vi "trialrunner.vi"() -> ()   [LabVIEW 2012]
uses:
  testing/log_event.ctl
  Experiment info.ctl
  testing/mode_conrols.ctl
  testing/ui_override_opts.ctl
  testing/control_selector.ctl
  initialization/micron_globals.vi
  <vilib>/Utility/xml.llb/Read From XML File(array).vi
panel:
  out "Actuate":bool
  out "Mode controls":T1
  in  "Allow skipping":bool
  in  "error in":errorcluster
  in  "Data path":string="c:\\data\\trials\\"
  out "Warning":bool
  out "Error":bool
  out "Retake":bool
  in  "Config name":string="trial"
  in  "Result data decimate":i32=5
  out "Start time":u32
  out "Prompt number":i32
  out "File exists":bool
  in  "Completed Trial Index":i32
  out "Information":string
  in  "New Experiment":bool
  out "Num Trials":i32
  in  "Back":bool
  in  "Next":bool
  in  "Subject Information":T2={" Subject"=-1, " Experiment"=1}
  in  "Trial Index":i32
  out "Trial status":T3[](array[typedef]) {"Timestamp" format="%<%.3X>T"}
  in  "Stop trial":bool caption="Stop"
  in  "Start":bool
  out "Run/stop":bool
  out "File name":path
  out "Save trace":bool
  in  "stop":bool
  # "Subject Information"
  # "Trial Management"
  # "m"
  # "Micron \nTrial \nManager"
  # "Authorized Personnel Only"
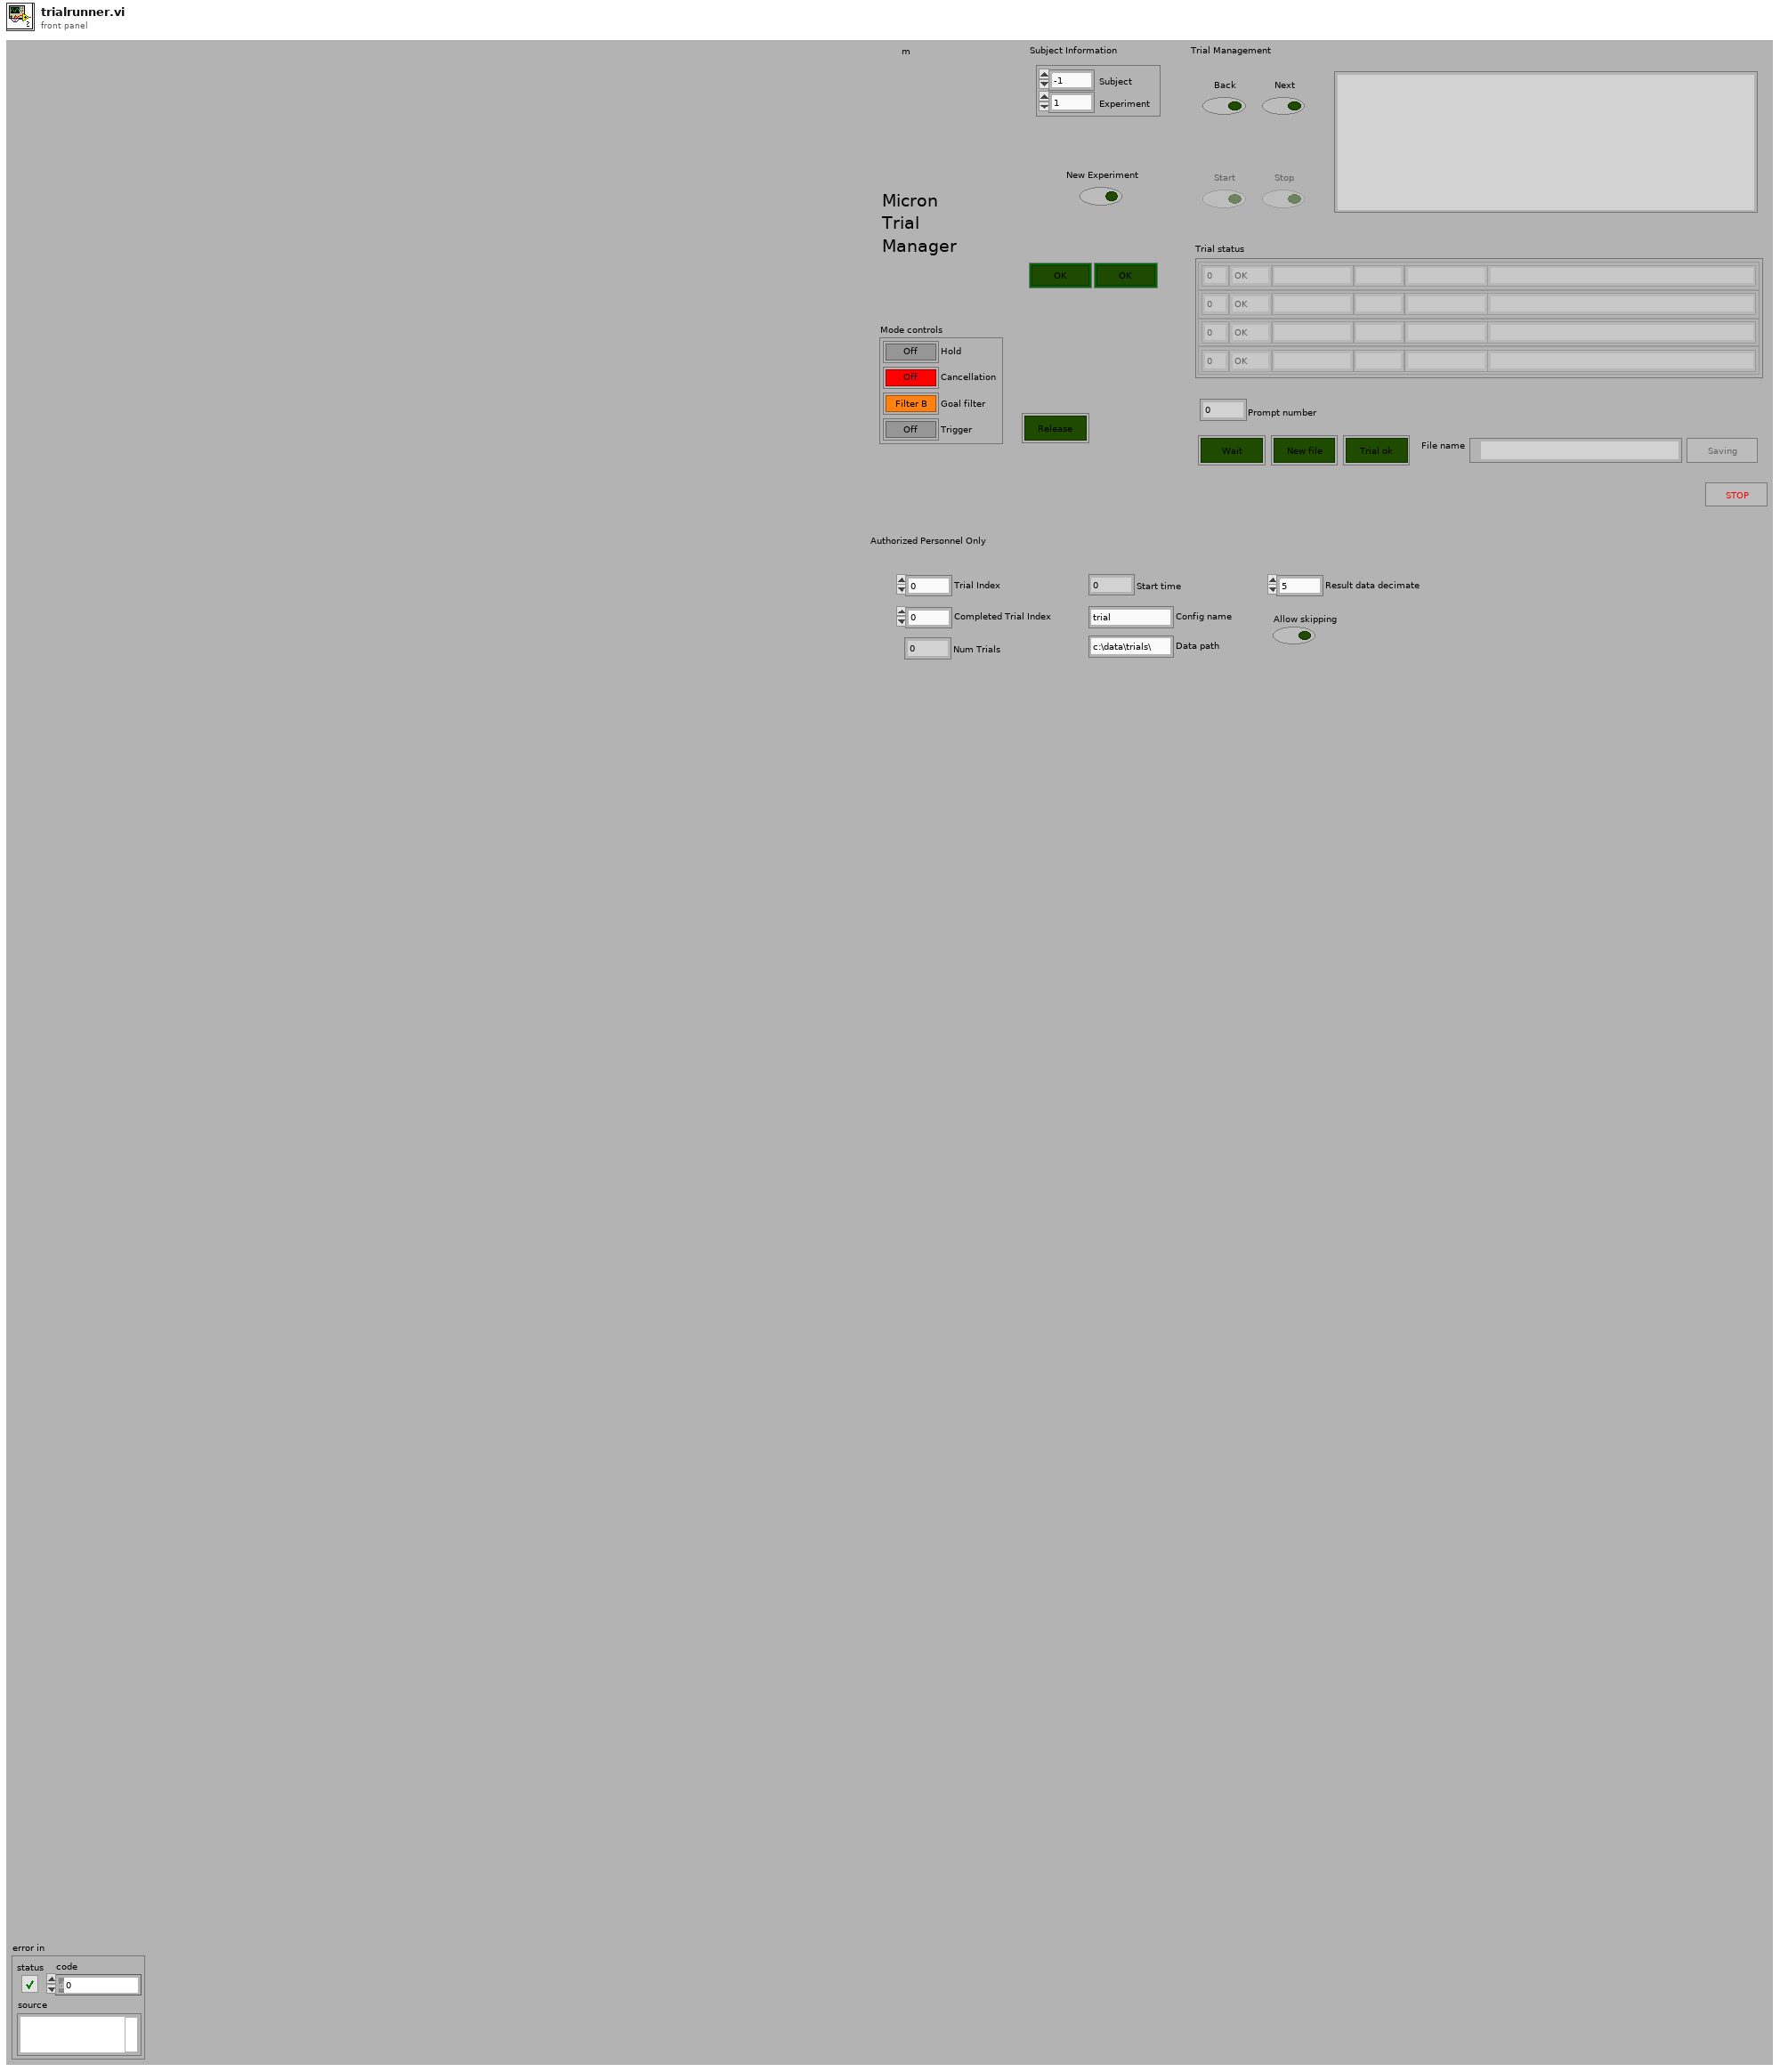
[diagram p1: front panel]
types:
  T1 = typedef "mode_conrols.ctl" = cluster{"Hold":bool, "Cancellation":bool, "Goal filter":bool, "Trigger":bool}
  T2 = typedef "Experiment info.ctl" = cluster{" Subject":i32, " Experiment":i32}
  T3 = typedef "log_event.ctl" = cluster{"Facility ID":i32, "Severity":enum16{"OK", "Debug", "Warn", "Error"}, "Timestamp":timestamp, "Facility":string, "State":string, "Message":string}
  T4 = typedef "ui_override_opts.ctl" = cluster{"Triggering":bool, "Parameters":bool, "Stimulus":bool, "Calibration":bool, "Modes":bool}
  T5 = typedef "Micron params.ctl" = cluster{"Stimulus":T6, "Goal Filter A":T8, "Mode controls":T1, "Manipulator type":enum16{"Current piezo", "Voltage piezo"}, "Manipulator calibration":T9, "Network":T11, "Goal Filter B":T8, "Cancellation":T12, "Transition time":sgl, "Estimation":T14}
  T6 = typedef "stimulus.ctl" = cluster{"Type":enum16{"Off", "Step", "Sine", "Triangle", "Arbitrary"}, "Phase":dbl, "Amplitude":sgl[], "Injection point":T7, "Closed loop":bool, "Offset":sgl[], "Tip -> world":bool, "Frequency":dbl, "Length":dbl}
  T7 = typedef "injection_point.ctl" = enum16{"Total pose", "V limiter", "Goal ", "Link position", "KF link position", "Inverse kin", "Link goal", "Link error", "Controller", "Output", "Drive", "Light"}
  T8 = typedef "goal_loop_parms.ctl" = cluster{"Speedup max":sgl, "Speedup thresh":sgl, "Speedup nonlin":sgl, "Filters":cluster{"Lower Fc":sgl, "Lower Q":sgl, "Scale factor":sgl, "Upper Fc":sgl, "Upper Q":sgl, "V limit":sgl, "V limit range":sgl}[]}
  T9 = typedef "manipulator_cal.ctl" = cluster{"Tool offsets":sgl[][], "Tip light calibration":T10, "Handle light calibration":T10, "Base pivots":sgl[][], "Output pivots":sgl[][], "Length center":sgl, "Workspace height":sgl[], "Workspace diameter":sgl[], "Linearization":sgl[][], "Stack travel":sgl, "Saturation pos":sgl, "Inverse filters":cluster{"filter structure":enum32{"IIR 2nd Order", "IIR 4th Order"}, "Reverse Coefficients":dbl[], "Forward Coefficients":dbl[]}[]}
  T10 = typedef "probe_calibration.ctl" = sgl[][]
  T11 = typedef "network_params.ctl" = cluster{"Remote Host":string, "Send Status":bool, "Send Port":u16, "Recv Commands":bool, "Recv Port":u16}
  T12 = typedef "sq_control_params.ctl" = cluster{"KP":T13, "KI":sgl, "KD":T13, "Max vel":sgl, "Max acc":sgl, "Int error limit":sgl, "RCM gain":sgl, "Bypass":bool, "Degraded gain":sgl}
  T13 = typedef "decoupled_gain.ctl" = cluster{"XY":sgl, "Rxy":sgl, "Z":sgl, "Rz":sgl}
  T14 = typedef "estimation_controls.ctl" = cluster{"Link":cluster{"Measure noise":dbl[], "Process noise":dbl[], "Alt process noise":dbl[], "Alt turnoff cycles":i32, "Innovation limit":dbl[], "Residue threshold":dbl, "Enable":bool}, "Handle":cluster{"Measure noise":dbl[], "Process noise":dbl[], "State limits":dbl[], "Innovation limit":dbl[], "Prediction Lookahead":sgl, "Enable":bool}}
  T15 = typedef "Rendezvous RefNum" = refnum<k1>
  T16 = typedef "control_selector.ctl" = cluster{"Selection":enum32{"No Selection", "Left", "Middle", "Right"}, "Mode":enum16{"Up", "Down", "Toggle", "Pulse", "Always", "Never"}}
  T17 = enum8{"Enabled", "Disabled", "Disabled and Grayed Out"}
  T18 = typedef "micron_config.ctl" = cluster{"rt fifo":refnum<k33>, "Analog output task":refnum<k21>, "Analog output task 2":refnum<k21>, "Stimulus AO task":refnum<k21>, "Low-rate AIN task":refnum<k21>, "Pedal out task":refnum<k21>, "Pedal in task":refnum<k21>, "Loop timing source":string, "Relay out task":refnum<k21>, "Send UDP Conn":refnum<k16>, "Recv UDP Conn":refnum<k16>, "Host Addr":dbl, "I2C interface":T19, "trace_start notifier":refnum<notifier>, "trace_done notifier":refnum<notifier>, "ASAP FIFO":refnum<k33>}
  T19 = typedef "i2c_interface.ctl" = cluster{"FPGA VI Reference":T20}
  T20 = typedef "fpga_reference.ctl" = refnum<k20>
  T21 = typedef "trial_condition.ctl" = cluster{"Type":enum16{"Undefined", "Start", "Normal", "Rest", "Done"}, "Task":u16, "Code":string, "Duration":dbl, "Prompts":u16, "Mode controls":T1, "Variable":bool, "Hold":bool}
  T22 = enum16{"Undefined", "Start", "Normal", "Rest", "Done"}
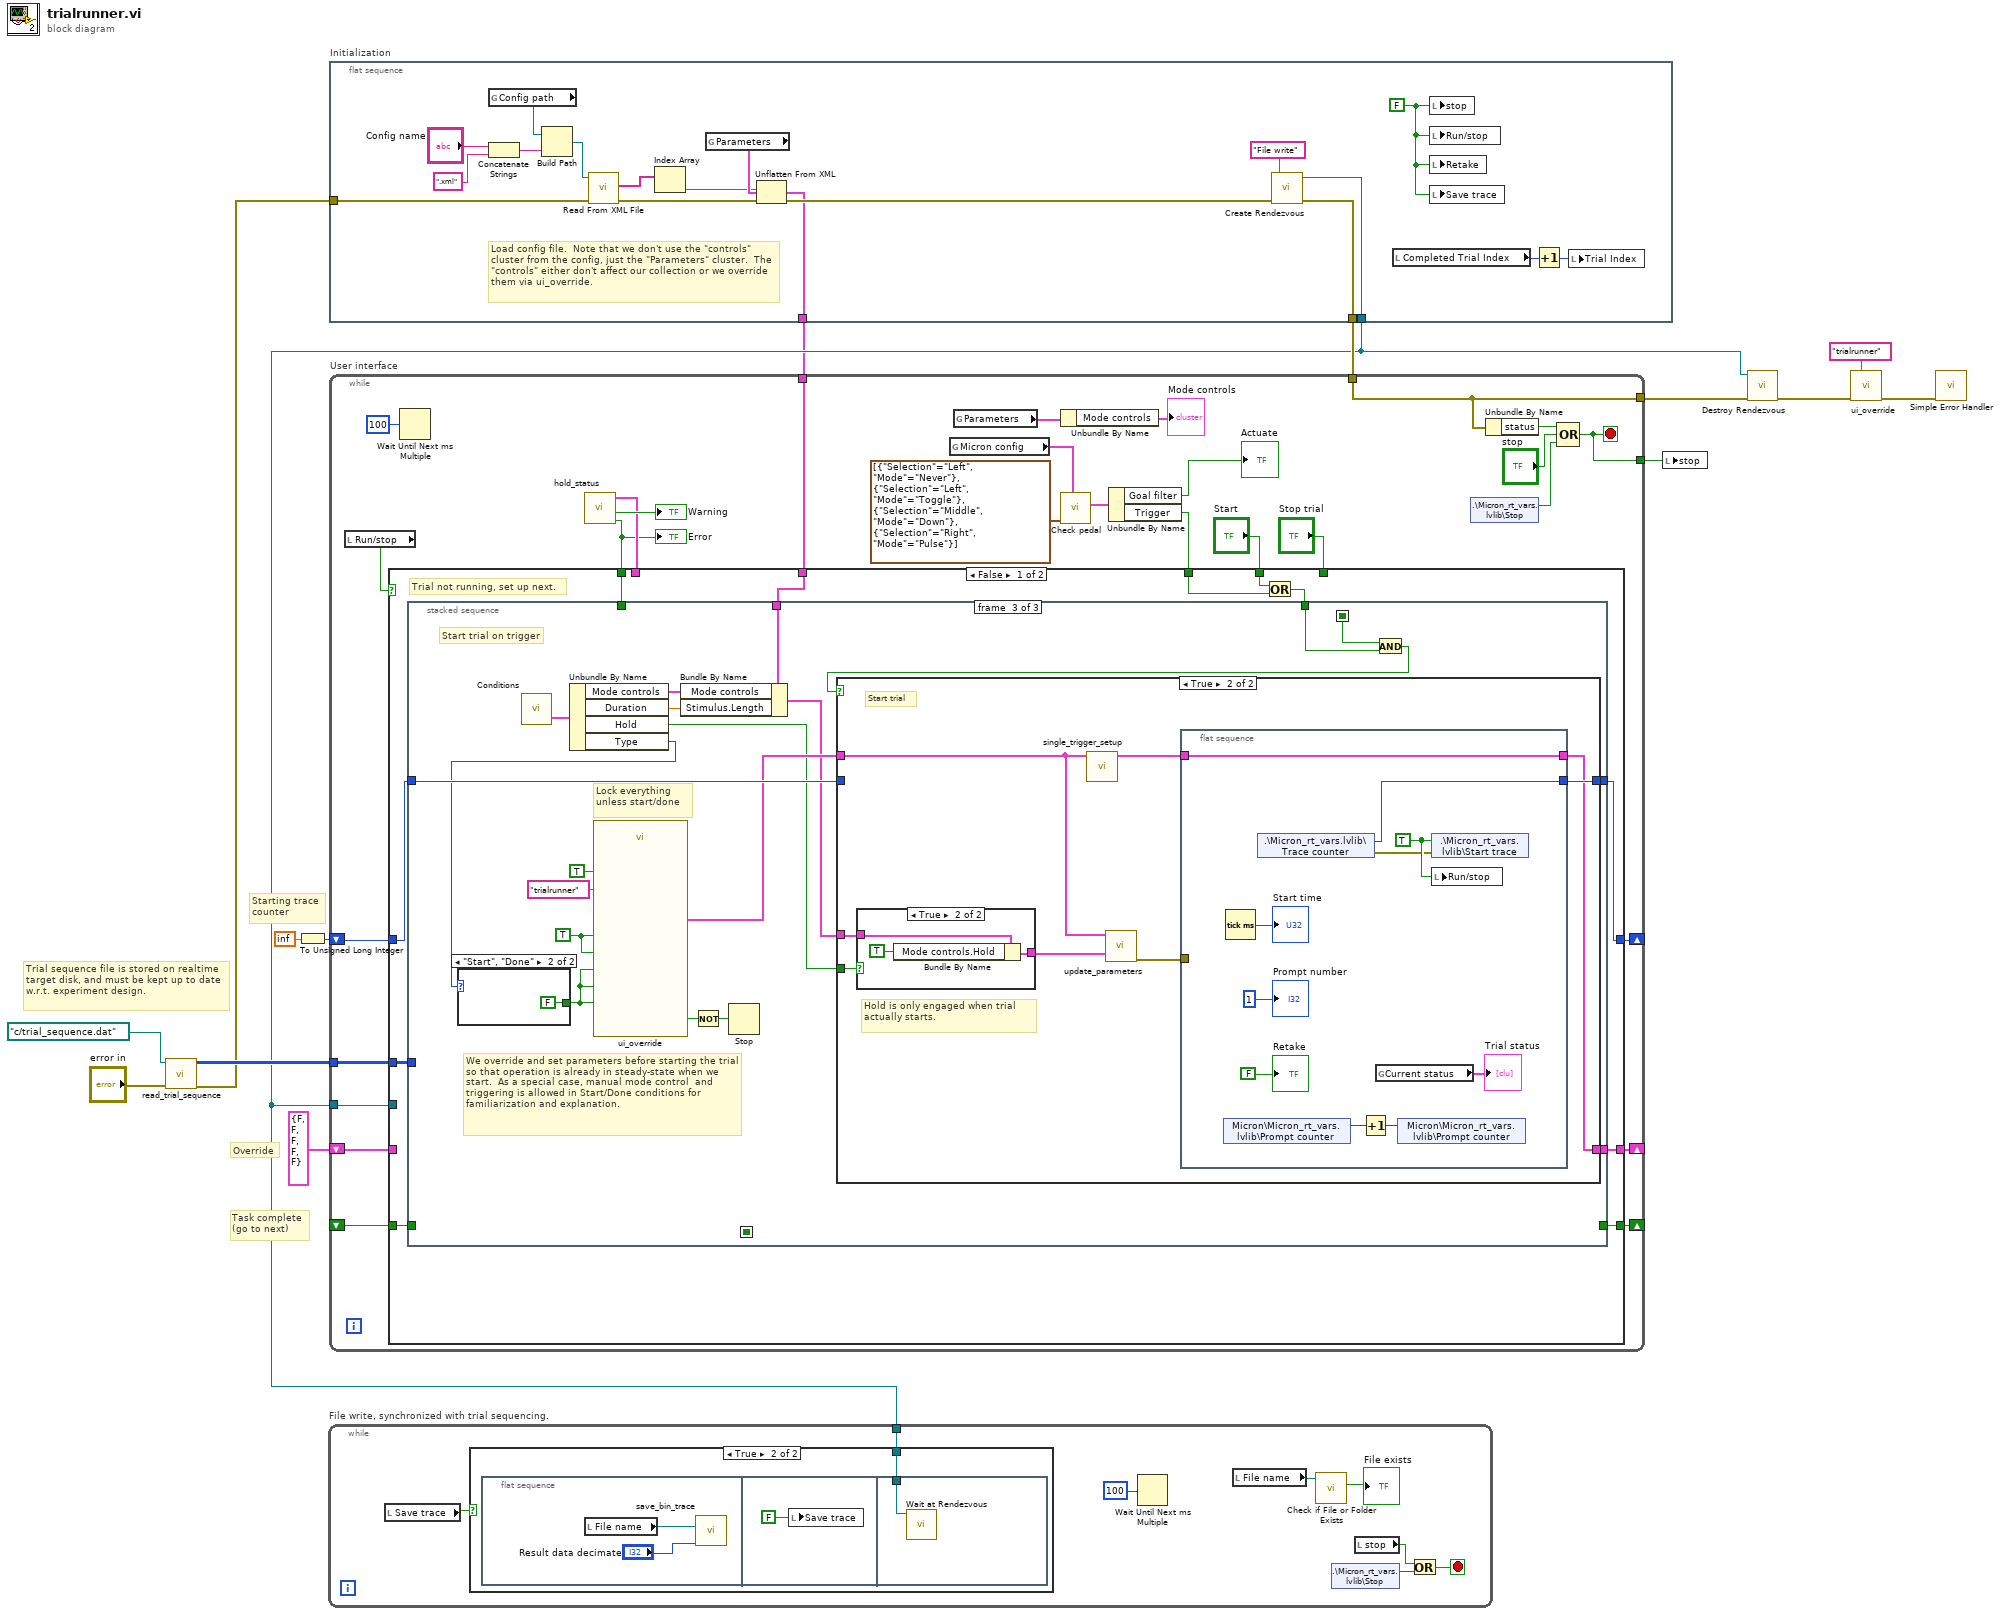
[diagram p0: block diagram]
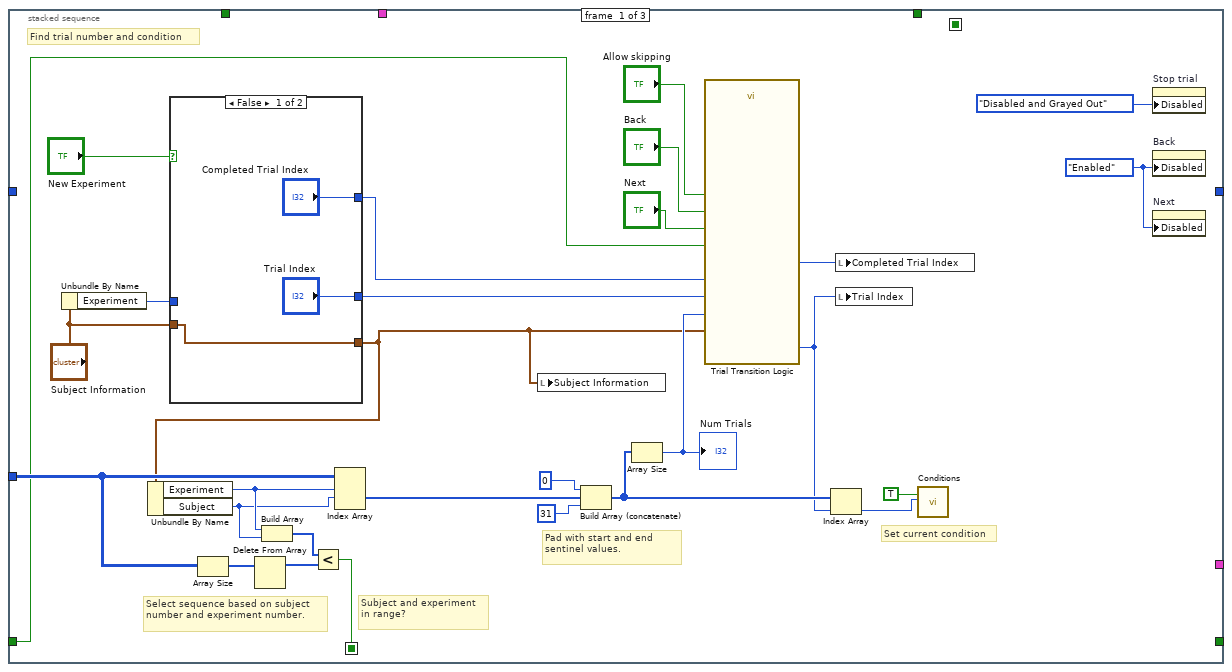
[diagram p2: hidden frame]
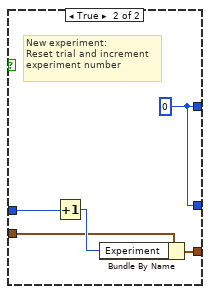
[diagram p3: hidden frame]
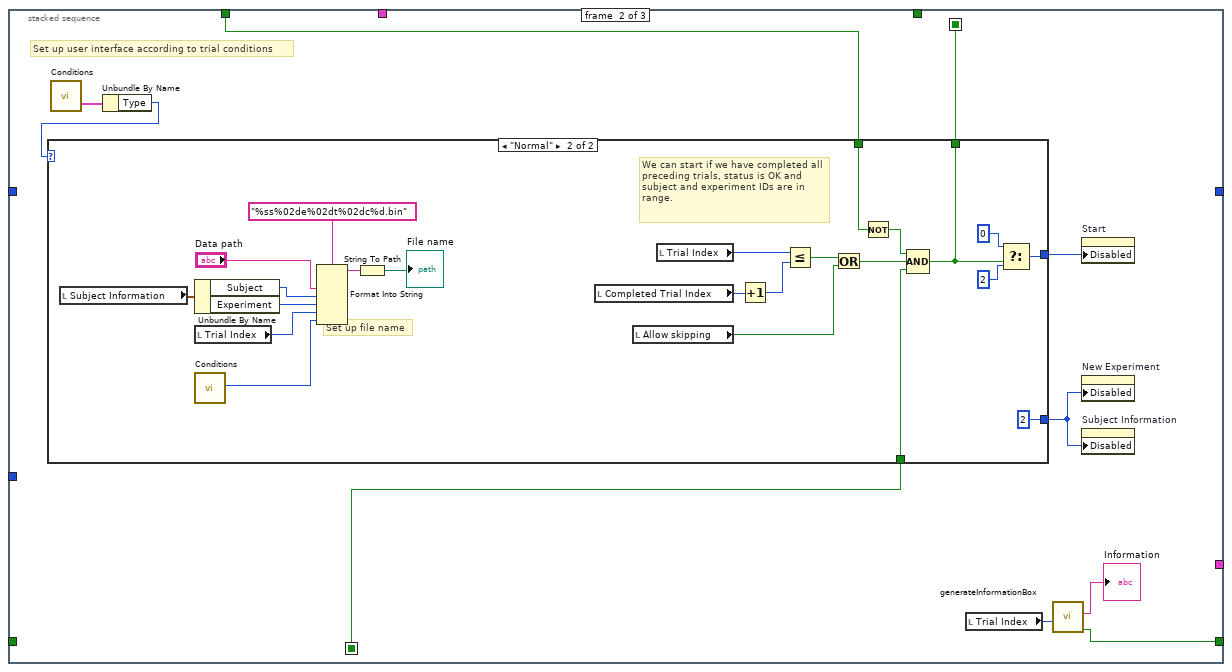
[diagram p4: hidden frame]
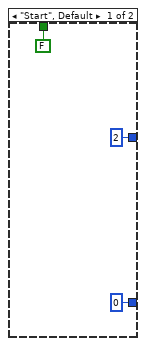
[diagram p5: hidden frame]
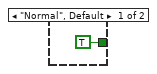
[diagram p6: hidden frame]
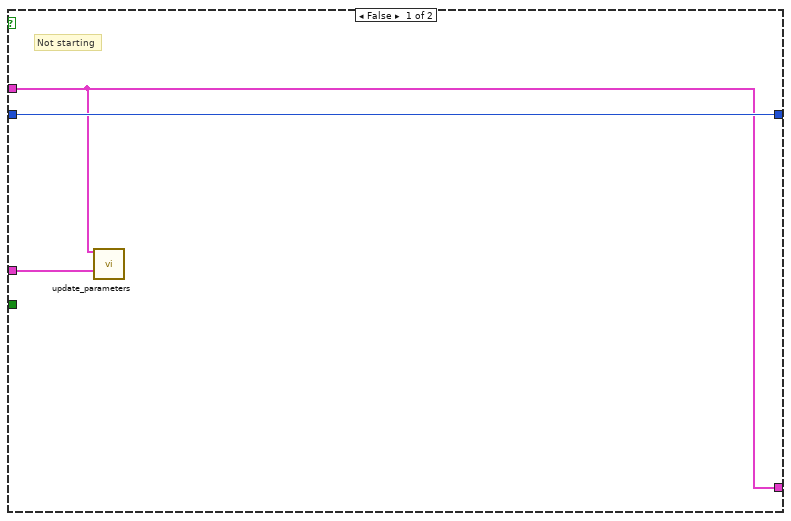
[diagram p7: hidden frame]
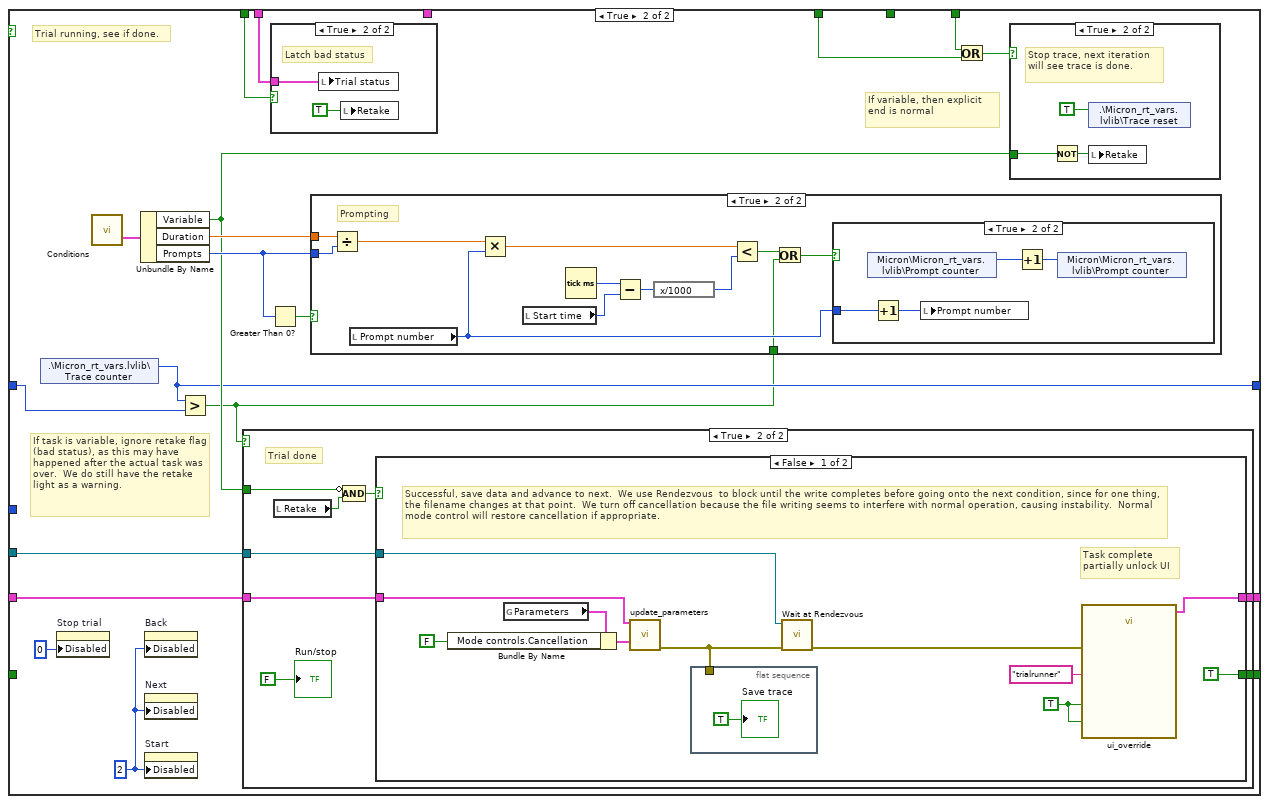
[diagram p9: hidden frame]
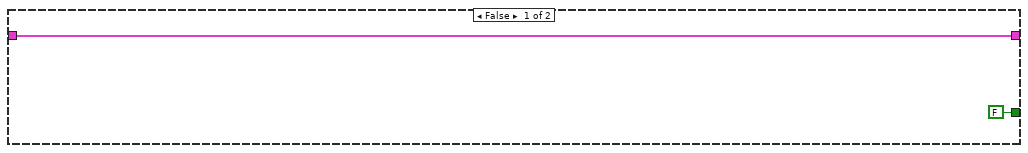
[diagram p13: hidden frame]
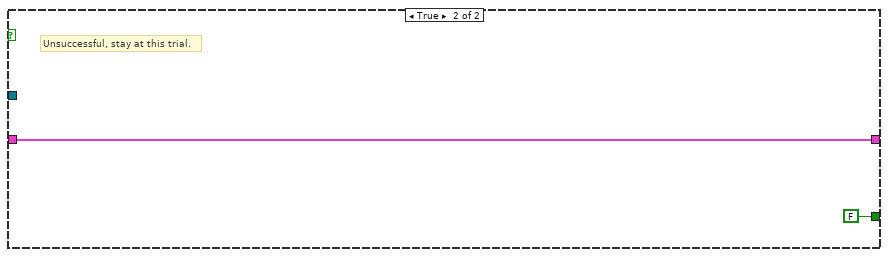
[diagram p14: hidden frame]
diagram:
  # "Override"
  # "Starting trace \ncounter"
  # "Task complete\n(go to next)"
  # "Trial sequence file is stored on realtime target disk, and must be kept up to date w.r.t. experiment design."
  n1 = call "read_trial_sequence.vi"("error in (no error)"="error in", "file path"=path "c:/trial_sequence.dat" ("file path (dialog if empty)")) -> ("error out"=w4:errorcluster, "Array"=w15:i32[][][])  [unwired: 8 in]
  n2 = To Unsigned Long Integer(number=inf) -> (unsigned 32bit integer=w1:u32)
  n3 = while "File write, synchronized with trial sequencing." {
    tunnel: w12 -> [w22]
    stop <- w16 stop-if-true
    n4 = local read "Save trace"() -> (w23:bool)
    n5 = case shown="True" w23 {
      tunnel: w22 -> [_ w24]
      frame False {
      }
      frame True {
        n6 = flat-sequence {
          tunnel: w24 -> [w28]
          frame #0 {
            n7 = local read "File name"() -> (w26:path)
            n8 = call "save_bin_trace.vi"("Decimate"="Result data decimate", "File path"=w26) -> ()  [unwired: 10 out]
          }
          frame #1 {
            n9 = local write "Save trace"(FALSE ("Save trace")) -> ()
          }
          frame #2 {
            n10 = call <vilib>:"Wait at Rendezvous.vi"("rendezvous"=w28) -> ()  [unwired: 2 in, 5 out]
          }
        }
      }
    }
    n11 = Wait Until Next ms Multiple(millisecond multiple=u32 100) -> ()  [unwired: 1 out]
    n12 = local read "File name"() -> (w20:path)
    n13 = call <vilib>:"Check if File or Folder Exists.vi"("path"=w20) -> ("file or folder exists?"=→"File exists":bool)  [unwired: 1 in, 9 out]
    n14 = shared-variable ".\\Micron_rt_vars.lvlib\\Stop"() -> (w18:bool)  [unwired: 2 out]
    n15 = local read "stop"() -> (w17:bool)
    n16 = Or(x=w17, y=w18) -> (x .or. y?=w16:bool)
  }
  n17 = flat-sequence "Initialization" {
    tunnel: [w45] -> w14
    tunnel: [w44] -> w12
    tunnel: [w31] -> w11
    tunnel: w4 -> [w29]
    frame #0 {
      w30 = FALSE ("Run/stop")
      # "Load config file.  Note that we don't use the \"controls\"  cluster from the config, just the \"Parameters\" cluster.  The \"controls\" either don't affect our collection or we override them via ui_override."
      n18 = global read "micron_globals.vi" "Config path"() -> (w39:path)
      n19 = Concatenate Strings("Config name", ".xml" ("string")) -> (w38:string)
      n20 = Build Path(base path=w39, name or relative path=w38) -> (appended path=w41:path)
      n21 = call-poly <vilib>:"Read From XML File.vi"("error in (no error)"=w29, "XML File Path"=w41) -> ("error out"=w33:errorcluster, "XML Elements"=w35:string[])  [unwired: 8 out]
      n22 = Index Array(array=w35) -> (element=w34:string)  [unwired: 1 in]
      n23 = global read "micron_globals.vi" "Parameters"() -> (w36:T5)
      n24 = Unflatten From XML(xml string=w34, type=w36, error in (no error)=w33) -> (value=w31:T5, error out=w32:errorcluster)
      n25 = call <vilib>:"Create Rendezvous.vi"("error in (no error)"=w32, "name (unnamed)"="File write") -> ("error out"=w45:errorcluster, "rendezvous"=w44:T15)  [unwired: 1 in, 3 out]
      n26 = local read "Completed Trial Index"() -> (w43:i32)
      n27 = local write "stop"(w30) -> ()
      n28 = local write "Run/stop"(w30) -> ()
      n29 = local write "Retake"(w30) -> ()
      n30 = local write "Save trace"(w30) -> ()
      n31 = Increment(x=w43) -> (x+1=w42:i32)
      n32 = local write "Trial Index"(w42) -> ()
    }
  }
  n33 = while "User interface" {
    tunnel: [w55] -> w13
    tunnel: w14 -> [w55]
    shift-right: [w69] -> _
    shift-left: w1 -> [w68]
    tunnel: w15 -> [w67]
    tunnel: w12 -> [w65]
    shift-right: [w63] -> _
    shift-left: _ -> [w62]
    tunnel: w11 -> [w58]
    shift-right: [w57] -> _
    shift-left: T4 {"Triggering"=FALSE, "Parameters"=FALSE, "Stimulus"=FALSE, "Calibration"=FALSE, "Modes"=FALSE} ("Override") -> [w56]
    tunnel: [w50] -> w7
    stop <- w50 stop-if-true
    n34 = local read "Run/stop"() -> (w71:bool)
    n35 = Wait Until Next ms Multiple(millisecond multiple=u32 100) -> ()  [unwired: 1 out]
    n36 = call "hold_status.vi"() -> ("Error"=w59:bool, "Warning"=→"Warning":bool, "Hold status"=w60:T3[])  [unwired: 9 in]
    "Error" <- w59
    n37 = global read "micron_globals.vi" "Micron config"() -> (w54:T18)
    n38 = global read "micron_globals.vi" "Parameters"() -> (w49:T5)
    n39 = Unbundle By Name(w49) -> ("Mode controls"=→"Mode controls":T1)
    n40 = call "Check pedal.vi"("Micron config"=w54, "Pedal selector"=T16[] [{"Selection"=enum."Left", "Mode"=enum."Never"}, {"Selection"=enum."Left", "Mode"=enum."Toggle"}, {"Selection"=enum."Middle", "Mode"=enum."Down"}, {"Selection"=enum."Right", "Mode"=enum."Pulse"}]) -> ("New mode controls"=w53:T1)  [unwired: 1 in, 8 out]
    n41 = Unbundle By Name(w53) -> ("Goal filter"=→"Actuate":bool, "Trigger"=w52:bool)
    n42 = case shown="False" w71 {
      tunnel: [w81 w206] -> w69
      tunnel: w68 -> [w78 w223]
      tunnel: "Start" -> [w83 _]
      tunnel: "Stop trial" -> [_ w220]
      tunnel: w67 -> [w85 _]
      tunnel: w52 -> [w84 w218]
      tunnel: w65 -> [_ w217]
      tunnel: [w80 w212] -> w63
      tunnel: w62 -> [w79 _]
      tunnel: w60 -> [_ w209]
      tunnel: w59 -> [w75 w210]
      tunnel: w58 -> [w77 _]
      tunnel: [w76 w207] -> w57
      tunnel: w56 -> [_ w208]
      frame False {
        # "Trial not running, set up next."
        n43 = Or(x=w83, y=w84) -> (x .or. y?=w82:bool)
        n44 = stacked-sequence {
          seq-local: [_ w124 _] -> [_ _ w177]
          seq-local: [w88 _ _] -> [_ w122 _]
          tunnel: w82 -> [_ _ w176]
          tunnel: w85 -> [w101 _ _]
          tunnel: [_ _ w174] -> w81
          tunnel: [_ w125 _] -> w80
          tunnel: w79 -> [w98 _ _]
          tunnel: w78 -> [_ _ w173]
          tunnel: w77 -> [_ _ w163]
          tunnel: [_ _ w172] -> w76
          tunnel: w75 -> [_ w123 _]
          frame #0 {
            w93 = T17."Enabled" ("Disabled")
            # "Subject and experiment in range?"
            # "Set current condition"
            # "Find trial number and condition"
            # "Pad with start and end sentinel values."
            # "Select sequence based on subject number and experiment number."
            n45 = Unbundle By Name("Subject Information") -> ("Experiment"=w104:i32)
            n46 = case shown="False" "New Experiment" {
              tunnel: w104 -> [_ w121]
              tunnel: "Subject Information" -> [w116 w119]
              tunnel: ["Trial Index" w117] -> w103
              tunnel: [w116 w118] -> w99
              tunnel: ["Completed Trial Index" w117] -> w96
              frame False {
              }
              frame True {
                w117 = 0 ("trialIndex")
                # "New experiment:\nReset trial and increment \nexperiment number"
                n47 = Increment(x=w121) -> (x+1=w120:i32)
                n48 = Bundle By Name(cluster=w119, "Experiment"=w120) -> (w118:T2)
              }
            }
            n49 = Unbundle By Name(w99) -> ("Experiment"=w92:i32, "Subject"=w87:i32)
            n50 = Array Size(array=w101) -> (size(s)=w91:i32[])
            n51 = Delete From Array(array=w91) -> (array with subset deleted=w90:i32[])  [unwired: 2 in, 1 out]
            n52 = Build Array(w92, w87) -> (w89:i32[])
            n53 = Less?(x=w89, y=w90) -> (x < y?=w88:bool)
            n54 = Index Array(array=w101, index (dim 0)=w92, index (dim 1)=w87) -> (element=w110:i32[])  [unwired: 1 in]
            n55 = local write "Subject Information"(w99) -> ()
            n56 = Build Array (concatenate)(0 ("element"), w110, 31 ("element")) -> (w107:i32[])
            n57 = Array Size(array=w107) -> (size(s)=w100:i32)
            "Num Trials" <- w100
            n58 = call "Trial Transition Logic.vi"("Completed Trial Index"=w96, "Allow skipping"="Allow skipping", "Old trial index"=w103, "Back"="Back", "Subject Information"=w99, "Num Trials"=w100, "Task complete"=w98, "Next"="Next") -> ("New Completed Trial Index"=w95:i32, "New trial index"=w102:i32)  [unwired: 2 out]
            n59 = Index Array(array=w107, index=w102) -> (element=w113:i32)
            n60 = local write "Completed Trial Index"(w95) -> ()
            n61 = local write "Trial Index"(w102) -> ()
            n62 = call "Conditions.vi"("Set current"=TRUE, "New condition code"=w113) -> ()  [unwired: 18 out]
            n63 = property on="Stop trial" class="Bool"("Disabled"=T17."Disabled and Grayed Out") -> ()  [unwired: 2 in, 2 out]
            n64 = property on="Back" class="Bool"("Disabled"=w93) -> ()  [unwired: 2 in, 2 out]
            n65 = property on="Next" class="Bool"("Disabled"=w93) -> ()  [unwired: 2 in, 2 out]
          }
          frame #1 {
            # "Set up user interface according to trial conditions"
            n66 = call "Conditions.vi"() -> ("Current condition"=w131:T21)  [unwired: 2 in, 17 out]
            n67 = Unbundle By Name(w131) -> ("Type"=w126:T22)
            n68 = case shown="\"Normal\"" w126 {
              tunnel: [u8 2 ("Disabled") w155] -> w130
              tunnel: [u8 0 ("Disabled") u8 2 ("Disabled")] -> w129
              tunnel: [FALSE w143] -> w124
              tunnel: w123 -> [_ w142]
              tunnel: w122 -> [_ w138]
              frame "Start", Default {
              }
              frame "Normal" {
                # "Set up file name"
                # "We can start if we have completed all preceding trials, status is OK and subject and experiment IDs are in range."
                n69 = local read "Subject Information"() -> (w150:T2)
                n70 = Unbundle By Name(w150) -> ("Subject"=w140:i32, "Experiment"=w145:i32)
                n71 = local read "Trial Index"() -> (w147:i32)
                n72 = call "Conditions.vi"() -> ("Condition code"=w148:i32)  [unwired: 2 in, 17 out]
                n73 = Format Into String(format string="%ss%02de%02dt%02dc%d.bin", "Data path", w140, w145, w147, w148) -> (resulting string=w149:string)  [unwired: 2 in, 1 out]
                n74 = String To Path(string=w149) -> (path=→"File name":path)
                n75 = local read "Completed Trial Index"() -> (w144:i32)
                n76 = local read "Allow skipping"() -> (w135:bool)
                n77 = local read "Trial Index"() -> (w153:i32)
                n78 = Increment(x=w144) -> (x+1=w154:i32)
                n79 = Less Or Equal?(x=w153, y=w154) -> (x <= y?=w137:bool)
                n80 = Or(x=w137, y=w135) -> (x .or. y?=w136:bool)
                n81 = Not(x=w142) -> (.not. x?=w141:bool)
                n82 = Compound Arithmetic op=AND(w141, w136, w138) -> (w143:bool)
                n83 = Select(t=u8 0, s=w143, f=u8 2 ("t")) -> (s? t:f=w155:u8)
              }
            }
            n84 = local read "Trial Index"() -> (w127:i32)
            n85 = call "generateInformationBox.vi"("Trial Index"=w127) -> ("Break over"=w125:bool, "Information Box"=→"Information":string)  [unwired: 4 in, 5 out]
            n86 = property on="Start" class="Bool"("Disabled"=w130) -> ()  [unwired: 2 in, 2 out]
            n87 = property on="New Experiment" class="Bool"("Disabled"=w129) -> ()  [unwired: 2 in, 2 out]
            n88 = property on="Subject Information" class="Clust (strict)"("Disabled"=w129) -> ()  [unwired: 2 in, 2 out]
          }
          frame #2 {
            w167 = TRUE ("Parameters")
            # "We override and set parameters before starting the trial so that operation is already in steady-state when we start.  As a special case, manual mode control  and triggering is allowed in Start/Done conditions for familiarization and explanation."
            # "Lock everything unless start/done"
            # "Start trial on trigger"
            n89 = call "Conditions.vi"() -> ("Current condition"=w166:T21)  [unwired: 2 in, 17 out]
            n90 = Unbundle By Name(w166) -> ("Mode controls"=w165:T1, "Duration"=w164:dbl, "Hold"=w158:bool, "Type"=w161:T22)
            n91 = case shown="\"Start\", \"Done\"" w161 {
              tunnel: [TRUE ("Parameters") FALSE ("Parameters")] -> w160
              frame "Normal", Default {
              }
              frame "Start", "Done" {
              }
            }
            n92 = call "ui_override.vi"("Triggering"=w160, "VI name"="trialrunner", "Parameters"=w167, "Stimulus"=w160, "Calibration"=w167, "All or nothing"=TRUE, "Modes"=w160) -> ("Override"=w162:T4, "Got all"=w170:bool)  [unwired: 6 in, 1 out]
            n93 = Bundle By Name(cluster=w163, "Mode controls"=w165, "Stimulus.Length"=w164) -> (w159:T5)
            n94 = Not(x=w170) -> (.not. x?=w171:bool)
            n95 = Stop(stop? (T)=w171) -> ()
            n96 = And(x=w177, y=w176) -> (x .and. y?=w175:bool)
            n97 = case shown="True" w175 {
              tunnel: [w182 w189] -> w174
              tunnel: w173 -> [w182 _]
              tunnel: [w181 w188] -> w172
              tunnel: w162 -> [w181 w184]
              tunnel: w159 -> [w180 w186]
              tunnel: w158 -> [_ w187]
              frame False {
                # "Not starting"
                n98 = call "update_parameters.vi"("Modify"=w181, "Parameters"=w180) -> ()  [unwired: 12 in, 2 out]
              }
              frame True {
                # "Hold is only engaged when trial actually starts."
                # "Start trial"
                n99 = case shown="True" w187 {
                  tunnel: w186 -> [w191 w194]
                  tunnel: [w191 w192] -> w185
                  frame False {
                  }
                  frame True {
                    n100 = Bundle By Name(cluster=w194, "Mode controls.Hold"=TRUE) -> (w192:T5)
                  }
                }
                n101 = call "single_trigger_setup.vi"("Override in"=w184) -> ("Override out"=w190:T4)  [unwired: 10 in]
                n102 = call "update_parameters.vi"("Modify"=w184, "Parameters"=w185) -> ("error out"=w183:errorcluster)  [unwired: 12 in, 1 out]
                n103 = flat-sequence {
                  tunnel: w190 -> [w195]
                  tunnel: [w197] -> w189
                  tunnel: [w195] -> w188
                  tunnel: w183 -> [_]
                  frame #0 {
                    w204 = TRUE ("Start trace")
                    n104 = shared-variable "Micron\\Micron_rt_vars.lvlib\\Prompt counter"() -> (w200:u32)  [unwired: 2 out]
                    n105 = Tick Count (ms)() -> (millisecond timer value=→"Start time":u32)
                    n106 = shared-variable ".\\Micron_rt_vars.lvlib\\Trace counter"() -> (w197:u32, error out=w196:errorcluster)  [unwired: 1 out]
                    n107 = Increment(x=w200) -> (x+1=w201:u32)
                    n108 = global read "micron_globals.vi" "Current status"() -> (→"Trial status":T3[])
                    n109 = shared-variable "Micron\\Micron_rt_vars.lvlib\\Prompt counter"(w201) -> ()  [unwired: 2 out]
                    n110 = shared-variable ".\\Micron_rt_vars.lvlib\\Start trace"(w204, error in=w196) -> ()  [unwired: 1 out]
                    n111 = local write "Run/stop"(w204) -> ()
                    "Prompt number" <- 1 ("Prompt number")
                    "Retake" <- FALSE ("Retake")
                  }
                }
              }
            }
          }
        }
      }
      frame True {
        w222 = u8 2 ("Disabled")
        # "If task is variable, ignore retake flag (bad status), as this may have happened after the actual task was over.  We do still have the retake light as a warning."
        # "If variable, then explicit end is normal"
        # "Trial running, see if done."
        n112 = shared-variable ".\\Micron_rt_vars.lvlib\\Trace counter"() -> (w206:u32)  [unwired: 2 out]
        n113 = property on="Stop trial" class="Bool"("Disabled"=u8 0) -> ()  [unwired: 2 in, 2 out]
        n114 = call "Conditions.vi"() -> ("Current condition"=w216:T21)  [unwired: 2 in, 17 out]
        n115 = Unbundle By Name(w216) -> ("Variable"=w211:bool, "Duration"=w215:dbl, "Prompts"=w213:u16)
        n116 = property on="Back" class="Bool"("Disabled"=w222) -> ()  [unwired: 2 in, 2 out]
        n117 = property on="Next" class="Bool"("Disabled"=w222) -> ()  [unwired: 2 in, 2 out]
        n118 = property on="Start" class="Bool"("Disabled"=w222) -> ()  [unwired: 2 in, 2 out]
        n119 = Greater?(x=w206, y=w223) -> (0:w205:bool)
        n120 = case shown="True" w205 {
          tunnel: w217 -> [_ w250]
          tunnel: [FALSE ("Save trace") w249] -> w212
          tunnel: w211 -> [_ w246]
          tunnel: w208 -> [w242 w245]
          tunnel: [w242 w244] -> w207
          frame False {
          }
          frame True {
            # "Trial done"
            n121 = local read "Retake"() -> (w248:bool)
            n122 = Compound Arithmetic op=AND(invert w246, w248) -> (w247:bool)
            n123 = case shown="False" w247 {
              tunnel: w250 -> [w262 _]
              tunnel: [TRUE ("Save trace") FALSE ("Save trace")] -> w249
              tunnel: w245 -> [w260 w264]
              tunnel: [w259 w264] -> w244
              frame False {
                w254 = TRUE ("Parameters")
                # "Task complete\npartially unlock UI"
                # "Successful, save data and advance to next.  We use Rendezvous  to block until the write completes before going onto the next condition, since for one thing, the filename changes at that point.  We turn off cancellation because the file writing seems to interfere with normal operation, causing instability.  Normal mode control will restore cancellation if appropriate."
                n124 = global read "micron_globals.vi" "Parameters"() -> (w258:T5)
                n125 = Bundle By Name(cluster=w258, "Mode controls.Cancellation"=FALSE) -> (w257:T5)
                n126 = call "update_parameters.vi"("Modify"=w260, "Parameters"=w257) -> ("error out"=w252:errorcluster)  [unwired: 12 in, 1 out]
                n127 = flat-sequence {
                  tunnel: w252 -> [_]
                  frame #0 {
                    "Save trace" <- TRUE ("Save trace")
                  }
                }
                n128 = call <vilib>:"Wait at Rendezvous.vi"("error in (no error)"=w252, "rendezvous"=w262) -> ("error out"=w253:errorcluster)  [unwired: 1 in, 4 out]
                n129 = call "ui_override.vi"("VI name"="trialrunner", "Parameters"=w254, "Calibration"=w254, "error in"=w253) -> ("Override"=w259:T4)  [unwired: 9 in, 2 out]
              }
              frame True {
                # "Unsuccessful, stay at this trial."
              }
            }
            "Run/stop" <- FALSE ("Run/stop")
          }
        }
        n130 = Greater Than 0?(x=w213) -> (x > 0?=w214:bool)
        n131 = case shown="True" w210 {
          tunnel: w209 -> [_ w241]
          frame False {
          }
          frame True {
            # "Latch bad status"
            n132 = local write "Trial status"(w241) -> ()
            n133 = local write "Retake"(TRUE ("Retake")) -> ()
          }
        }
        n134 = case shown="True" w214 {
          tunnel: w215 -> [_ w232]
          tunnel: w213 -> [_ w231]
          tunnel: w205 -> [_ w224]
          frame False {
          }
          frame True {
            # "Prompting"
            n135 = Divide(x=w232, y=w231) -> (x/y=w230:dbl)
            n136 = local read "Prompt number"() -> (w227:i32)
            n137 = Multiply(x=w230, y=w227) -> (x*y=w229:dbl)
            n138 = local read "Start time"() -> (w233:u32)
            n139 = Tick Count (ms)() -> (millisecond timer value=w234:u32)
            n140 = Subtract(x=w234, y=w233) -> (x-y=w235:u32)
            n141 = expression code="x/1000"(w235) -> (w228:u32)
            n142 = Less?(x=w229, y=w228) -> (x < y?=w226:bool)
            n143 = Or(x=w226, y=w224) -> (x .or. y?=w225:bool)
            n144 = case shown="True" w225 {
              tunnel: w227 -> [_ w239]
              frame False {
              }
              frame True {
                n145 = shared-variable "Micron\\Micron_rt_vars.lvlib\\Prompt counter"() -> (w236:u32)  [unwired: 2 out]
                n146 = Increment(x=w239) -> (x+1=w238:i32)
                n147 = local write "Prompt number"(w238) -> ()
                n148 = Increment(x=w236) -> (x+1=w237:u32)
                n149 = shared-variable "Micron\\Micron_rt_vars.lvlib\\Prompt counter"(w237) -> ()  [unwired: 2 out]
              }
            }
          }
        }
        n150 = Or(x=w220, y=w218) -> (x .or. y?=w219:bool)
        n151 = case shown="True" w219 {
          tunnel: w211 -> [_ w266]
          frame False {
          }
          frame True {
            # "Stop trace, next iteration will see trace is done."
            n152 = Not(x=w266) -> (.not. x?=w267:bool)
            n153 = shared-variable ".\\Micron_rt_vars.lvlib\\Trace reset"(TRUE ("Start trace")) -> ()  [unwired: 2 out]
            n154 = local write "Retake"(w267) -> ()
          }
        }
      }
    }
    n155 = shared-variable ".\\Micron_rt_vars.lvlib\\Stop"() -> (w72:bool)  [unwired: 2 out]
    n156 = Unbundle By Name(w55) -> ("status"=w74:bool)
    n157 = Compound Arithmetic op=OR(w74, "stop", w72) -> (w50:bool)
  }
  n158 = local write "stop"(w7) -> ()
  n159 = call <vilib>:"Destroy Rendezvous.vi"("error in (no error)"=w13, "rendezvous"=w12) -> ("error out"=w9:errorcluster)  [unwired: 5 out]
  n160 = call "ui_override.vi"("VI name"="trialrunner", "error in"=w9) -> ("error out"=w8:errorcluster)  [unwired: 11 in, 2 out]
  n161 = call <vilib>:"Simple Error Handler.vi"("error in (no error)"=w8) -> ()  [unwired: 1 in, 8 out]
